vi "PIM Measure Key Array.vi"(4 "Conversion":enum16{"Cluster - HTML", "HTML - Cluster"}(ring), 6 "PIM Test Parameters":T1={"Stimulus"={"C1 Pwr dBm"=0.0, "C2 Pwr dBm"=0.0, "Power Units"=enum."dBm", "Meas Type"=enum."Time", "C1 Freq MHz"=0.0, "C2 Freq MHz"=0.0, "Swept Freq Step"=0}, "Measure"={"IM Order"=0, "Direction"=0, "Averaging"=1, "ALC ON?"=TRUE, "Peak Hold?"=TRUE, "Peak last N"=1, "Ref Level dBm"=-100.0, "Ref Units"=enum."dBm", "Num Samples"=1, "Sample units"=enum."Sample(s)", "Update Rate (s)"=0.0, "DUT PORT"=enum."Port 1", "Percent (%)"=100}, "Display"={"Power Scale"={"yRange_min"=0, "yRange_max"=0}, "xRange_span"=5}} {"Stimulus"."Swept Freq Step" items=[".2", ".4", "1.0", "2.0"]; "Measure"."Averaging" items=["None", "Minimum", "Normal", "High", "Maximum"]; "Measure"."Direction" items=["Reverse", "Forward", "Auxiliary"]; "Measure"."IM Order" items=["3rd", "5th", "7th", "9th", "11th", "13th", "15th", "17th", "19th", "21st", "23rd", "25th", "27th", "29th", "31st", "33rd"]}, 7 "Key Array In":T11) -> (1 "PIM Test Parameters (out)":T1={"Stimulus"={"C1 Pwr dBm"=0.0, "C2 Pwr dBm"=0.0, "Power Units"=enum."dBm", "Meas Type"=enum."Time", "C1 Freq MHz"=0.0, "C2 Freq MHz"=0.0, "Swept Freq Step"=0}, "Measure"={"IM Order"=0, "Direction"=0, "Averaging"=1, "ALC ON?"=TRUE, "Peak Hold?"=TRUE, "Peak last N"=1, "Ref Level dBm"=-100.0, "Ref Units"=enum."dBm", "Num Samples"=1, "Sample units"=enum."Sample(s)", "Update Rate (s)"=0.0, "DUT PORT"=enum."Port 1", "Percent (%)"=100}, "Display"={"Power Scale"={"yRange_min"=0, "yRange_max"=0}, "xRange_span"=5}} {"Stimulus"."Swept Freq Step" items=[".2", ".4", "1.0", "2.0"]; "Measure"."Averaging" items=["None", "Minimum", "Normal", "High", "Maximum"]; "Measure"."Direction" items=["Reverse", "Forward", "Auxiliary"]; "Measure"."IM Order" items=["3rd", "5th", "7th", "9th", "11th", "13th", "15th", "17th", "19th", "21st", "23rd", "25th", "27th", "29th", "31st", "33rd"]}, 2 "Key Array Out":T11)   [LabVIEW 2011]
uses:
  ITK/utils/keyedarr.llb/Keyed Array.ctl
  TypeDefs/PIM Test Parameters.ctl
  TypeDefs/PIM Stimulus Parameters.ctl
  BPIMCore/HW IO/PIM Sweep Step Size.ctl
  TypeDefs/PIM Measurement Parameters.ctl
  BPIMCore/HW IO/IMOrder.ctl
  BPIMCore/HW IO/MeasMode.ctl
  BPIMCore/HW IO/HW Averaging.ctl
  TypeDefs/PIM Meas Units.ctl
  BPIMCore/HW IO/DUTport.ctl
  TypeDefs/PIM Display Parameters.ctl
  ITK/utils/strutil.llb/Case Matching.ctl
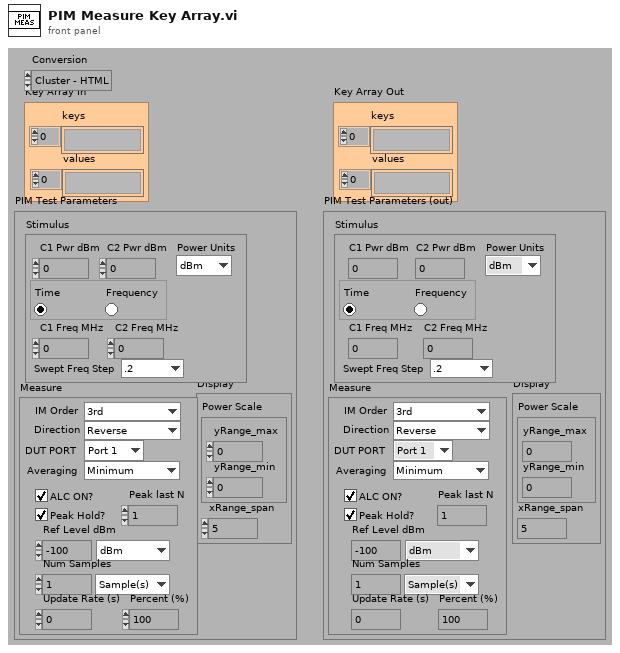
[diagram p1: front panel]
types:
  T1 = typedef "PIM Test Parameters.ctl" = cluster{"Stimulus":T2, "Measure":T4, "Display":T10}
  T2 = typedef "PIM Stimulus Parameters.ctl" = cluster{"C1 Pwr dBm":dbl, "C2 Pwr dBm":dbl, "Power Units":enum16{"dBm", "Watts"}, "Meas Type":enum32{"Time", "Frequency"}, "C1 Freq MHz":dbl, "C2 Freq MHz":dbl, "Swept Freq Step":T3}
  T3 = typedef "PIM Sweep Step Size.ctl" = u16
  T4 = typedef "PIM Measurement Parameters.ctl" = cluster{"IM Order":T5, "Direction":T6, "Averaging":T7, "ALC ON?":bool, "Peak Hold?":bool, "Peak last N":u32, "Ref Level dBm":dbl, "Ref Units":enum16{"dBm", "dBc"}, "Num Samples":u32, "Sample units":T8, "Update Rate (s)":dbl, "DUT PORT":T9, "Percent (%)":u8}
  T5 = typedef "IMOrder.ctl" = u8
  T6 = typedef "MeasMode.ctl" = u16
  T7 = typedef "HW Averaging.ctl" = u16
  T8 = typedef "PIM Meas Units.ctl" = enum16{"Sample(s)", "Second(s)", "Sweep(s)"}
  T9 = typedef "DUTport.ctl" = enum16{"Port 1", "Port 2"}
  T10 = typedef "PIM Display Parameters.ctl" = cluster{"Power Scale":cluster{"yRange_min":i32, "yRange_max":i32}, "xRange_span":u32}
  T11 = typedef "Keyed Array.ctl" = cluster{"keys":string[], "values":string[]}
  T12 = typedef "Case Matching.ctl" = enum16{"a != A", "a == A", "system"}
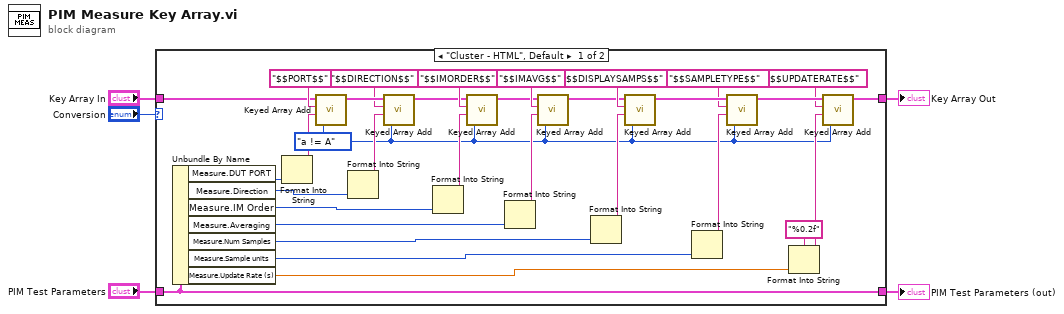
[diagram p0: block diagram]
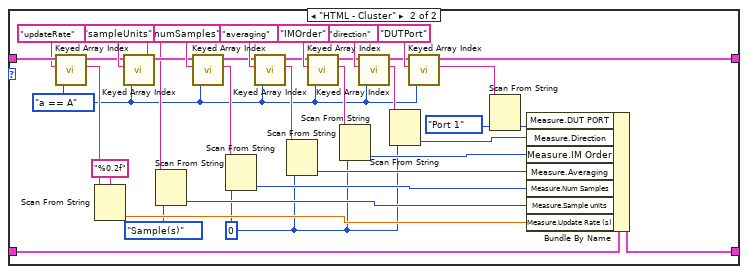
[diagram p2: hidden frame]
diagram:
  n1 = case shown="\"Cluster - HTML\", Default" "Conversion" {
    tunnel: "Key Array In" -> [w34 w73]
    tunnel: "PIM Test Parameters" -> [w12 w71]
    tunnel: [w24 w48] -> w3
    tunnel: [w12 w70] -> w2
    frame "Cluster - HTML", Default {
      w7 = Case_Matching."a != A" ("case matching (sensitive)")
      n2 = Unbundle By Name(w12) -> ("Measure.DUT PORT"=w23:T9, "Measure.Direction"=w21:T6, "Measure.IM Order"=w19:T5, "Measure.Averaging"=w11:T7, "Measure.Num Samples"=w16:u32, "Measure.Sample units"=w10:T8, "Measure.Update Rate (s)"=w14:dbl)
      n3 = Format Into String(w23) -> (resulting string=w22:string)  [unwired: 3 in, 1 out]
      n4 = call "Keyed Array Add.vi"("case matching (sensitive)"=w7, "value"=w22, "key"="$$PORT$$", "array in"=w34) -> ("array out"=w37:T11)  [unwired: 3 out]
      n5 = Format Into String(w21) -> (resulting string=w20:string)  [unwired: 3 in, 1 out]
      n6 = call "Keyed Array Add.vi"("case matching (sensitive)"=w7, "value"=w20, "key"="$$DIRECTION$$", "array in"=w37) -> ("array out"=w30:T11)  [unwired: 3 out]
      n7 = Format Into String(w19) -> (resulting string=w18:string)  [unwired: 3 in, 1 out]
      n8 = call "Keyed Array Add.vi"("case matching (sensitive)"=w7, "value"=w18, "key"="$$IMORDER$$", "array in"=w30) -> ("array out"=w32:T11)  [unwired: 3 out]
      n9 = Format Into String(w11) -> (resulting string=w17:string)  [unwired: 3 in, 1 out]
      n10 = call "Keyed Array Add.vi"("case matching (sensitive)"=w7, "value"=w17, "key"="$$IMAVG$$", "array in"=w32) -> ("array out"=w25:T11)  [unwired: 3 out]
      n11 = Format Into String(w16) -> (resulting string=w15:string)  [unwired: 3 in, 1 out]
      n12 = call "Keyed Array Add.vi"("case matching (sensitive)"=w7, "value"=w15, "key"="$$DISPLAYSAMPS$$", "array in"=w25) -> ("array out"=w28:T11)  [unwired: 3 out]
      n13 = Format Into String(w10) -> (resulting string=w9:string)  [unwired: 3 in, 1 out]
      n14 = call "Keyed Array Add.vi"("case matching (sensitive)"=w7, "value"=w9, "key"="$$SAMPLETYPE$$", "array in"=w28) -> ("array out"=w26:T11)  [unwired: 3 out]
      n15 = Format Into String(format string="%0.2f", w14) -> (resulting string=w13:string)  [unwired: 2 in, 1 out]
      n16 = call "Keyed Array Add.vi"("case matching (sensitive)"=w7, "value"=w13, "key"="$$UPDATERATE$$", "array in"=w26) -> ("array out"=w24:T11)  [unwired: 3 out]
    }
    frame "HTML - Cluster" {
      w40 = 0
      w38 = Case_Matching."a == A" ("case matching (sensitive)")
      n17 = call "Keyed Array Index.vi"("case matching (sensitive)"=w38, "key"="updateRate", "array in"=w73) -> ("value"=w51:string, "duplicate array"=w50:T11)  [unwired: 1 in, 2 out]
      n18 = Scan From String(format string="%0.2f", input string=w51) -> (output 1=w49:dbl)  [unwired: 2 in, 4 out]
      n19 = call "Keyed Array Index.vi"("case matching (sensitive)"=w38, "key"="sampleUnits", "array in"=w50) -> ("value"=w46:string, "duplicate array"=w52:T11)  [unwired: 1 in, 2 out]
      n20 = Scan From String(input string=w46, default 1=PIM_Meas_Units."Sample(s)" ("Measure.Sample units")) -> (output 1=w44:T8)  [unwired: 3 in, 3 out]
      n21 = call "Keyed Array Index.vi"("case matching (sensitive)"=w38, "key"="numSamples", "array in"=w52) -> ("value"=w43:string, "duplicate array"=w42:T11)  [unwired: 1 in, 2 out]
      n22 = Scan From String(input string=w43, default 1=w40) -> (output 1=w55:i32)  [unwired: 3 in, 3 out]
      n23 = call "Keyed Array Index.vi"("case matching (sensitive)"=w38, "key"="averaging", "array in"=w42) -> ("value"=w59:string, "duplicate array"=w57:T11)  [unwired: 1 in, 2 out]
      n24 = Scan From String(input string=w59, default 1=w40) -> (output 1=w56:i32)  [unwired: 3 in, 3 out]
      n25 = call "Keyed Array Index.vi"("case matching (sensitive)"=w38, "key"="IMOrder", "array in"=w57) -> ("value"=w61:string, "duplicate array"=w62:T11)  [unwired: 1 in, 2 out]
      n26 = Scan From String(input string=w61, default 1=w40) -> (output 1=w60:i32)  [unwired: 3 in, 3 out]
      n27 = call "Keyed Array Index.vi"("case matching (sensitive)"=w38, "key"="direction", "array in"=w62) -> ("value"=w64:string, "duplicate array"=w65:T11)  [unwired: 1 in, 2 out]
      n28 = Scan From String(input string=w64, default 1=w40) -> (output 1=w41:i32)  [unwired: 3 in, 3 out]
      n29 = call "Keyed Array Index.vi"("case matching (sensitive)"=w38, "key"="DUTPort", "array in"=w65) -> ("value"=w68:string, "duplicate array"=w48:T11)  [unwired: 1 in, 2 out]
      n30 = Scan From String(input string=w68, default 1=DUTport."Port 1" ("Measure.DUT PORT")) -> (output 1=w69:T9)  [unwired: 3 in, 3 out]
      n31 = Bundle By Name(cluster=w71, "Measure.DUT PORT"=w69, "Measure.Direction"=w41, "Measure.IM Order"=w60, "Measure.Averaging"=w56, "Measure.Num Samples"=w55, "Measure.Sample units"=w44, "Measure.Update Rate (s)"=w49) -> (w70:T1)
    }
  }
  "Key Array Out" <- w3
  "PIM Test Parameters (out)" <- w2
